vi "Load Class by Name.vi"(5 "Class Type":refnum<class>, 8 "error in (no error)":errorcluster, 11 "Class Name":string) -> (0 "error out":errorcluster, 1 "Success?":bool, 3 "Loaded Class":refnum<class>)   [LabVIEW 2020, in "ClassLoader.lvlib"]
uses:
  ClassLoader.lvlib
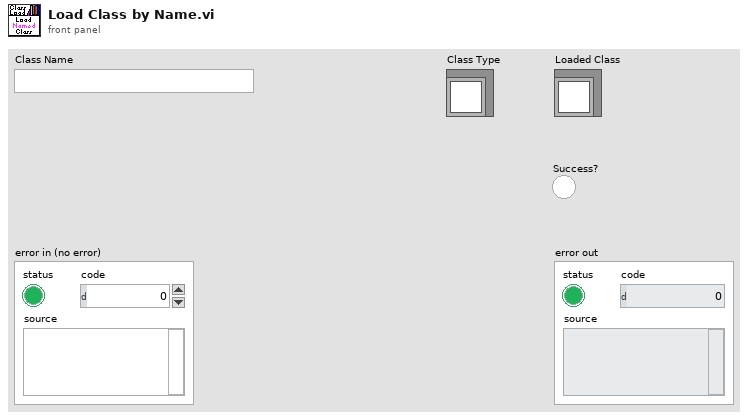
[diagram p1: front panel]
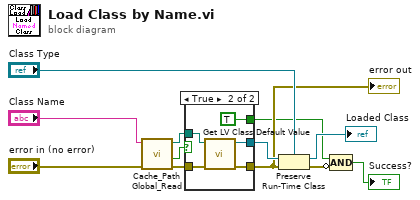
[diagram p0: block diagram]
diagram:
  n1 = call "Cache_Path Global_Read.vi"("error in (no error)"="error in (no error)", "Class Name"="Class Name") -> ("error out"=w4:errorcluster, "Success?"=w2:bool, "Class Path"=w1:path)  [unwired: 7 in]
  n2 = case shown="True" w2 {
    tunnel: w1 -> [_ w18]
    tunnel: [_ w17] -> w12
    tunnel: w4 -> [w13 w16]
    tunnel: [w13 w15] -> w9
    tunnel: [_ TRUE] -> w8
    frame False {
    }
    frame True {
      n3 = call <vilib>:"Get LV Class Default Value.vi"("error in (no error)"=w16, "class path"=w18) -> ("error out"=w15:errorcluster, "object"=w17:refnum<class>)  [unwired: 8 in]
    }
  }
  "error out" <- w9
  n4 = Preserve Run-Time Class(object in=w12, error in=w9, 2:"Class Type") -> (object out=→"Loaded Class":refnum<class>, error out=w7:errorcluster)
  n5 = Compound Arithmetic op=AND(w8, invert w7) -> (→"Success?":bool)
